vi "Inward Local Transition.vi"(7 "Timeout Period in ms (-1, never)":i32=-1, 8 "error in (no error)":errorcluster, 9 "Target State":refnum<class "State.lvclass">, 10 "Context in":refnum<class "Context.lvclass">, 11 "State in":refnum<class "State.lvclass">) -> (0 "error out":errorcluster, 2 "Context out":refnum<class "Context.lvclass">, 3 "State out":refnum<class "State.lvclass">)   [LabVIEW 2024, in "State.lvlib" / "State.lvclass"]
uses:
  State.lvclass
  Context/Context/Context.lvclass
  Container State/Container State.lvclass
  State.lvclass/State.ctl
  C:/Users/uspoaotto/OneDrive - Oregon Tool/Desktop/working copies/stateMachineActor/src/State Machine/State/State/State.lvclass
  C:/Users/uspoaotto/OneDrive - Oregon Tool/Desktop/working copies/stateMachineActor/src/State Machine/State/Container State/Container State.lvclass
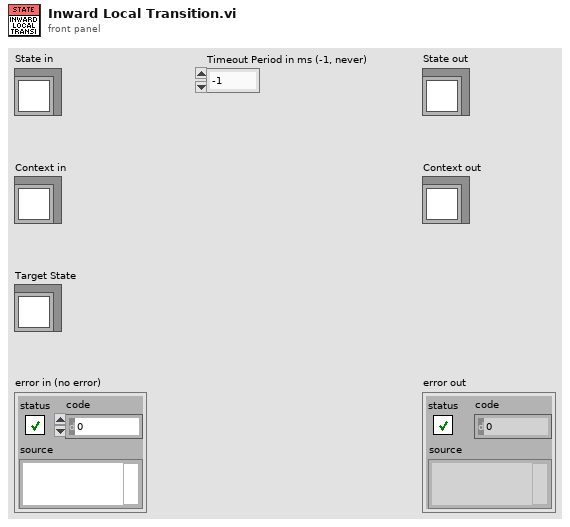
[diagram p1: front panel]
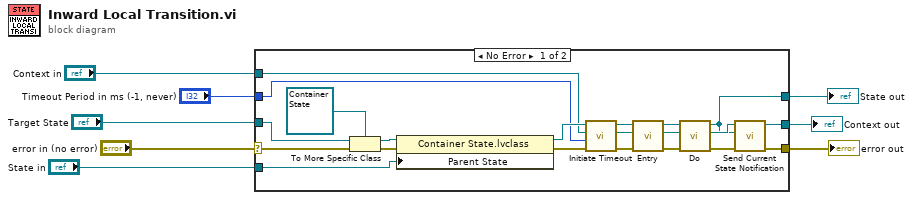
[diagram p0: block diagram]
diagram:
  n1 = case shown="No Error" "error in (no error)" {
    selector: "error in (no error)" -> [w24 w32]
    tunnel: [w17 w32] -> w7
    tunnel: [w19 w31] -> w5
    tunnel: "State in" -> [w21 w31]
    tunnel: [w16 w30] -> w2
    tunnel: "Target State" -> [w25 _]
    tunnel: "Context in" -> [w13 w30]
    tunnel: "Timeout Period in ms (-1, never)" -> [w11 _]
    frame No Error {
      n2 = To More Specific Class(target class=refnum<class "Container State.lvclass"> refnum ("State.lvlib:Container State.lvclass"), reference=w25, error in=w24) -> (specific class reference=w22:refnum<class "Container State.lvclass">, error out=w23:errorcluster)
      n3 = property class="Container State.lvclass"(reference=w22, error in=w23, "Parent State"=w21) -> (reference out=w15:refnum<class "Container State.lvclass">, error out=w10:errorcluster)
      n4 = call "Initiate Timeout.vi"("error in (no error)"=w10, "Timeout Period in ms (-1, never)"=w11, "Context in"=w13, "State in"=w15) -> ("error out"=w9:errorcluster, "Context out"=w12:refnum<class "Context.lvclass">, "State out"=w14:refnum<class "Container State.lvclass">)  [unwired: 5 in]
      n5 = call-dynamic "Entry.vi"("error in (no error)"=w9, "Context in"=w12, "State in"=w14) -> ("error out"=w27:errorcluster, "Context out"=w28:refnum<class "Context.lvclass">, "State out"=w29:refnum<class "Container State.lvclass">)  [unwired: 6 in]
      n6 = call-dynamic "Do.vi"("error in (no error)"=w27, "Context in"=w28, "State in"=w29) -> ("error out"=w18:errorcluster, "Context out"=w20:refnum<class "Context.lvclass">, "State out"=w19:refnum<class "Container State.lvclass">)  [unwired: 6 in]
      n7 = call "Send Current State Notification.vi"("error in (no error)"=w18, "State"=w19, "Context in"=w20) -> ("error out"=w17:errorcluster, "Context out"=w16:refnum<class "Context.lvclass">)  [unwired: 7 in]
    }
    frame Error {
    }
  }
  "error out" <- w7
  "State out" <- w5
  "Context out" <- w2
